vi "KI6221.vi"() -> ()   [LabVIEW 2025] (continued)
                                frame False {
                                }
                                frame True {
                                n821 = while {
                                tunnel: w1577 -> [w1593]
                                tunnel: w1576 -> [w1592]
                                tunnel: w1575 -> [w1588]
                                shift-right: [w1582] -> w1573
                                shift-left: w1574 -> [w1583]
                                tunnel: w1572 -> [w1581]
                                i -> [w1589]
                                stop <- w1586 stop-if-true
                                n822 = Increment(x=w1589) -> (x+1=w1587:i32)
                                n823 = call "VISAreadWrite.vi"("error in (no error)"=w1581, "GPIB INDEX Array"=i32[] [47], "GPIB ARRAY"=w1592, "VISA REFERENCE"=w1593) -> ("error out 15"=→"error out 38":errorcluster, "Read Buffer Array"=w1585:string[])
                                n824 = Greater Or Equal?(x=w1587, y=w1588) -> (x >= y?=w1586:bool)
                                n825 = Index Array(array=w1585, index=1) -> (element=w1579:string)
                                n826 = String Subset(string=w1579, length (rest)=254 ("length (rest)")) -> (substring=w1578:string)  [unwired: 1 in]
                                n827 = Concatenate Strings(w1583, w1578) -> (w1582:string)
                                }
                                }
                                }
                                n828 = String Subset(string=w1541, length (rest)=254 ("length (rest)")) -> (substring=w1540:string)  [unwired: 1 in]
                                n829 = Concatenate Strings(w1540, w1544) -> (w1545:string)
                                n830 = Spreadsheet String To Array(delimiter (Tab)=",", format string="%e", spreadsheet string=w1545, array type (2D Dbl)=dbl[] []) -> (array=w1563:dbl[])
                                n831 = while {
                                tunnel: w1563 -> [w1612]
                                shift-right: [w1611] -> w1556
                                shift-left: string[][] [] -> [w1607]
                                tunnel: w1561 -> [w1600]
                                tunnel: w1560 -> [w1601]
                                tunnel: w1558 -> [w1599]
                                tunnel: w1557 -> [w1598]
                                i -> [w1603]
                                stop <- w1622 stop-if-true
                                w1617 = "," ("delimiter (Tab)")
                                n832 = case shown="0, Default" w1599 {
                                tunnel: w1603 -> [w1625 w1636]
                                tunnel: w1601 -> [w1626 w1634]
                                tunnel: w1600 -> [w1627 w1633]
                                tunnel: [w1623 w1631] -> w1595
                                tunnel: w1598 -> [_ w1628]
                                frame 0, Default {
                                n833 = Multiply(x=w1625, y=w1627) -> (x*y=w1624:dbl)
                                n834 = Add(x=w1626, y=w1624) -> (x+y=w1623:dbl)
                                }
                                frame 1 {
                                n835 = Logarithm Base 10(1:w1634) -> (0:w1630:dbl)
                                n836 = case shown="True" w1628 {
                                tunnel: w1630 -> [w1638 w1639]
                                tunnel: [w1637 w1639] -> w1629
                                frame False {
                                n837 = Negate(x=w1638) -> (-x=w1637:dbl)
                                }
                                frame True {
                                }
                                }
                                n838 = Multiply(x=w1633, y=w1636) -> (x*y=w1632:dbl)
                                n839 = Add(x=w1629, y=w1632) -> (x+y=w1635:dbl)
                                n840 = Power Of 10(x=w1635) -> (10^x=w1631:dbl)
                                }
                                }
                                n841 = Index Array(array=w1612, index=w1603) -> (element=w1605:dbl)
                                n842 = Array Size(array=w1607) -> (size(s)=w1609:i32[])
                                n843 = Index Array(array=w1609, index=0) -> (element=w1606:i32)
                                n844 = Increment(x=w1606) -> (x+1=w1602:i32)
                                n845 = Array Size(array=w1612) -> (size(s)=w1610:i32)
                                n846 = Number To Engineering String(4:w1605) -> (0:w1614:string)  [unwired: 3 in]
                                n847 = Greater Or Equal?(x=w1602, y=w1610) -> (x >= y?=w1622:bool)
                                n848 = Number To Decimal String(number=w1603) -> (decimal integer string=w1616:string)  [unwired: 1 in]
                                n849 = Number To Exponential String(number=w1595, precision (6)=i16 3) -> (E-format string=w1597:string)  [unwired: 2 in]
                                n850 = Fract/Exp String To Number(string=w1597) -> (number=w1594:dbl)  [unwired: 3 in, 1 out]
                                n851 = Divide(x=w1605, y=w1594) -> (x/y=w1604:dbl)
                                n852 = Number To Engineering String(4:w1594) -> (0:w1615:string)  [unwired: 3 in]
                                n853 = Number To Engineering String(4:w1604) -> (0:w1613:string)  [unwired: 3 in]
                                n854 = Concatenate Strings(w1616, w1617, w1615, w1617, w1614, w1617, w1613) -> (w1618:string)
                                n855 = Spreadsheet String To Array(delimiter (Tab)=w1617, format string="%s", spreadsheet string=w1618, array type (2D Dbl)=string[] []) -> (array=w1619:string[])
                                n856 = Insert Into Array(array=w1607, index (row)=w1603, new element=w1619) -> (w1611:string[][])  [unwired: 1 in]
                                }
                                "I Sweep V Measure Data" <- w1556
                                n857 = Array Subset(array=w1556, index (col)=2 ("index"), length (col)=1 ("length")) -> (w1553:string[][])  [unwired: 2 in]
                                n858 = Fract/Exp String To Number(string=w1553) -> (number=w1552:dbl[][])  [unwired: 3 in, 1 out]
                                n859 = Array Max & Min(array=w1552) -> (max value=w1551:dbl)  [unwired: 3 out]
                                n860 = Greater?(x=w1551, y=1e+36) -> (0:w1549:bool)
                                n861 = call "Volt range problem"("Enable"=w1549) -> ()  [unwired: 9 in, 2 out]
                                }
                                }
                                "error out 19" <- w1527
                              }
                            }
                          }
                        }
                        n862 = local write "ABORT SWEEP"(w1425) -> ()
                      }
                      frame True {
                        # "INSTR Missing"
                        n863 = call "LOG error"("Enable"=w1682) -> ()  [unwired: 9 in, 2 out]
                        n864 = Build Array(w1685, w1684, w1683) -> (w1687:bool[])
                        n865 = Boolean Array To Number(Boolean array=w1687) -> (number=w1686:u32)
                        n866 = case shown="3" w1686 {
                          tunnel: w1685 -> [_ w1688 _ _ _ w1691 _ _]
                          tunnel: w1684 -> [_ _ w1689 _ _ _ w1692 _]
                          frame 0, Default {
                          }
                          frame 1 {
                            n867 = call "No 6220/6221 responding"("Enable"=w1688) -> ()  [unwired: 9 in, 2 out]
                          }
                          frame 2 {
                            n868 = call "No 2182/2182A responding"("Enable"=w1689) -> ()  [unwired: 9 in, 2 out]
                          }
                          frame 3 {
                            n869 = call "No Instruments Responding"() -> ()  [unwired: 10 in, 2 out]
                          }
                          frame 4 {
                            n870 = property on="Number of sweep points" class="DigNum (strict)"("Key Focus"=TRUE) -> ()  [unwired: 2 in, 2 out]
                            n871 = call "Too Many Points"() -> ()  [unwired: 10 in, 2 out]
                          }
                          frame 5 {
                            n872 = call "No 6220/6221 responding"("Enable"=w1691) -> ()  [unwired: 9 in, 2 out]
                          }
                          frame 6 {
                            n873 = call "No 2182/2182A responding"("Enable"=w1692) -> ()  [unwired: 9 in, 2 out]
                          }
                          frame 7 {
                            n874 = call "No Instruments Responding"() -> ()  [unwired: 10 in, 2 out]
                          }
                        }
                      }
                    }
                  }
                }
                n875 = local read "enable measure"() -> (w1331:bool)
                n876 = Not Equal?(x="enable measure LAST", y=w1331) -> (x != y?=w1333:bool)
                n877 = case shown="True" w1333 {
                  tunnel: w1331 -> [_ w1358]
                  frame False {
                  }
                  frame True {
                    n878 = case shown="False" w1358 {
                      tunnel: [u8 2 ("Disabled") u8 0 ("Disabled")] -> w1359
                      frame False {
                      }
                      frame True {
                      }
                    }
                    n879 = local write "enable measure LAST"(w1358) -> ()
                    n880 = property on="delta tabs 2" class="TabCtl (strict)"("Disabled"=w1359) -> ()  [unwired: 2 in, 2 out]
                  }
                }
                n881 = Not Equal?(x="X Axis:", y="X Axis: LAST") -> (x != y?=w1338:bool)
                n882 = Not Equal?(x="Y Axis:", y="Y Axis:  LAST") -> (x != y?=w1337:bool)
                n883 = Or(x=w1338, y=w1337) -> (x .or. y?=w1336:bool)
                n884 = case shown="True" w1336 {
                  tunnel: "Y Axis:" -> [_ w1364]
                  tunnel: "X Axis:" -> [_ w1365]
                  frame False {
                  }
                  frame True {
                    n885 = local write "Y Axis:  LAST"(w1364) -> ()
                    n886 = local write "X Axis: LAST"(w1365) -> ()
                    n887 = property on="X Axis:" class="Ring (strict)"() -> ("Strings []"=w1367:string[])  [unwired: 2 in, 2 out]
                    n888 = property on="Y Axis:" class="Ring (strict)"() -> ("Strings []"=w1366:string[])  [unwired: 2 in, 2 out]
                    n889 = local read "I Sweep V Measure Data"() -> (w1371:string[][])
                    n890 = Index Array(array=w1367, index=w1365) -> (element=w1363:string)
                    n891 = Index Array(array=w1366, index=w1364) -> (element=w1362:string)
                    n892 = Index Array(array=w1371, index (col)=w1365) -> (element=w1369:string[])  [unwired: 1 in]
                    n893 = Index Array(array=w1371, index (col)=w1364) -> (element=w1370:string[])  [unwired: 1 in]
                    n894 = Fract/Exp String To Number(string=w1369) -> (number=w1373:dbl[])  [unwired: 3 in, 1 out]
                    n895 = call "Convert to Dynamic Data6"("Array"=w1373) -> ("Dynamic Data Type"=w1374:dynamicdata)  [unwired: 3 in]
                    n896 = Fract/Exp String To Number(string=w1370) -> (number=w1375:dbl[])  [unwired: 3 in, 1 out]
                    n897 = call "Convert to Dynamic Data12"("Array"=w1375) -> ("Dynamic Data Type"=w1368:dynamicdata)  [unwired: 3 in]
                    n898 = call "Build XY Graph4"("Y Input"=w1368, "X Input"=w1374) -> ("XY Graph"=→"I Sweep Graph":cluster{"Y":dbl[], "Y":dbl[]}[])  [unwired: 8 in, 1 out]
                    n899 = property on="I Sweep Graph" class="XYGraph (strict)"("X Scale.Name Label.Text"=w1363, "Y Scale.Name Label.Text"=w1362) -> ()  [unwired: 2 in, 2 out]
                  }
                }
                n900 = local read "ABORT SWEEP"() -> (w1330:bool)
                n901 = Not(x=w1322) -> (.not. x?=w1323:bool)
                n902 = And(x=w1330, y=w1323) -> (x .and. y?=w1324:bool)
                n903 = case shown="True" w1324 {
                  tunnel: w1329 -> [_ w1354]
                  tunnel: w1328 -> [_ w1353]
                  frame False {
                  }
                  frame True {
                    w1350 = TRUE ("Page Selector Visible")
                    n904 = property on="ABORT SWEEP" class="Bool (strict)"("Disabled"=u8 2, "Value"=FALSE ("ABORT SWEEP")) -> ()  [unwired: 2 in, 2 out]
                    n905 = property on="RUN SWEEP" class="Bool"("Disabled"=u8 0) -> ()  [unwired: 2 in, 2 out]
                    n906 = call "VISAreadWrite.vi"("GPIB INDEX Array"=i32[] [36], "GPIB ARRAY"=w1353, "VISA REFERENCE"=w1354) -> ("error out 15"=→"error out 36":errorcluster)  [unwired: 1 in, 1 out]
                    n907 = property on="Basic Source" class="TabCtl (strict)"("Page Selector Visible"=w1350) -> ()  [unwired: 2 in, 2 out]
                    n908 = property on="Main Tabs" class="TabCtl (strict)"("Page Selector Visible"=w1350) -> ()  [unwired: 2 in, 2 out]
                  }
                }
              }
              frame "AC Source" {
                n909 = local write "Source TABS LAST"(w1710) -> ()
                n910 = Not(x=w1702) -> (.not. x?=w1699:bool)
                n911 = And(x="RUN 2", y=w1699) -> (x .and. y?=w1701:bool)
                n912 = local write "waveform tabs 2"("Waveform Type") -> ()
                n913 = local read "6220 VISA"() -> (w1707:refnum<visa-resource-name>)
                n914 = local read "GPIB Array"() -> (w1706:string[])
                n915 = case shown="True" w1701 {
                  tunnel: "Waveform Type" -> [_ w1721]
                  tunnel: w1706 -> [_ w1786]
                  tunnel: w1707 -> [_ w1785]
                  tunnel: [FALSE w1765] -> w1703
                  frame False {
                  }
                  frame True {
                    w1766 = u8 2 ("Disabled")
                    w1767 = 2.0 ("y")
                    # "amplitude"
                    # "offset"
                    # "NOT 6221"
                    n916 = property on="RUN 2" class="Bool"("Disabled"=u8 2) -> ()  [unwired: 2 in, 2 out]
                    n917 = call "VISAreadWrite.vi"("GPIB INDEX Array"=i32[] [0], "GPIB ARRAY"=w1786, "VISA REFERENCE"=w1785) -> ("error out 15"=→"error out 22":errorcluster, "Read Buffer Array"=w1790:string[])  [unwired: 1 in]
                    n918 = property on="Waveform Type" class="Ring (strict)"("Disabled"=w1766) -> ()  [unwired: 2 in, 2 out]
                    n919 = property on="waveform tabs 2" class="TabCtl (strict)"("Disabled"=w1766) -> ()  [unwired: 2 in, 2 out]
                    n920 = Add(x="Ramp from: (Amps)", y="Ramp to: (Amps)") -> (x+y=w1770:dbl)
                    n921 = Subtract(x="Ramp from: (Amps)", y="Ramp to: (Amps)") -> (x-y=w1768:dbl)
                    n922 = Index Array(array=w1790, index=1) -> (element=w1792:string)
                    n923 = Divide(x=w1770, y=w1767) -> (x/y=w1764:dbl)
                    n924 = property on="STOP 2" class="Bool"("Disabled"=u8 0) -> ()  [unwired: 2 in, 2 out]
                    n925 = Divide(x=w1768, y=w1767) -> (x/y=w1769:dbl)
                    n926 = Equal?(x="Ramp from: (Amps)", y="Ramp to: (Amps)") -> (x = y?=w1720:bool)
                    n927 = Absolute Value(x=w1769) -> (abs(x)=w1763:dbl)
                    n928 = Match Pattern(string=w1792, regular expression="MODEL 6221") -> (offset past match=w1789:i32)  [unwired: 1 in, 3 out]
                    n929 = Equal?(x=w1789, y=-1) -> (x = y?=w1727:bool)
                    n930 = property on="Voltage\n Compliance" class="DigNum (strict)"("Disabled"=w1766) -> ()  [unwired: 2 in, 2 out]
                    n931 = Number To Exponential String(number="Duty Cycle (%)") -> (E-format string=w1778:string)  [unwired: 3 in]
                    n932 = Number To Exponential String(number=w1764) -> (E-format string=w1780:string)  [unwired: 3 in]
                    n933 = Number To Exponential String(number=w1763) -> (E-format string=w1779:string)  [unwired: 3 in]
                    n934 = property on="Signal Repetition \nFrequency (Hz)" class="DigNum (strict)"("Disabled"=w1766) -> ()  [unwired: 2 in, 2 out]
                    n935 = Equal?(x=w1721, y=0) -> (x = y?=w1722:bool)
                    n936 = And(x=w1720, y=w1722) -> (x .and. y?=w1719:bool)
                    n937 = Add(x="Offset (Amps)", y="Amplitude (Amps)") -> (x+y=w1756:dbl)
                    n938 = Subtract(x="Offset (Amps)", y="Amplitude (Amps)") -> (x-y=w1755:dbl)
                    n939 = Add(x=w1764, y=w1763) -> (x+y=w1762:dbl)
                    n940 = Subtract(x=w1764, y=w1763) -> (x-y=w1761:dbl)
                    n941 = Greater?(x=w1756, y=0.105) -> (0:w1751:bool)
                    n942 = Less?(x=w1755, y=-0.105) -> (x < y?=w1752:bool)
                    n943 = Greater?(x=w1762, y=0.105) -> (0:w1740:bool)
                    n944 = Less?(x=w1761, y=-0.105) -> (x < y?=w1758:bool)
                    n945 = Or(x=w1751, y=w1752) -> (x .or. y?=w1732:bool)
                    n946 = Number To Exponential String(number="Amplitude (Amps)") -> (E-format string=w1777:string)  [unwired: 3 in]
                    n947 = Number To Exponential String(number="Duty Cycle (%)") -> (E-format string=w1775:string)  [unwired: 3 in]
                    n948 = Number To Exponential String(number="Offset (Amps)") -> (E-format string=w1776:string)  [unwired: 3 in]
                    n949 = Or(x=w1740, y=w1758) -> (x .or. y?=w1734:bool)
                    n950 = Equal?(x=w1721, y=0) -> (x = y?=w1733:bool)
                    n951 = And(x=w1734, y=w1733) -> (x .and. y?=w1730:bool)
                    n952 = Equal?(x=w1721, y=1) -> (x = y?=w1731:bool)
                    n953 = And(x=w1732, y=w1731) -> (x .and. y?=w1729:bool)
                    n954 = Add(x="Offset (Amps)", y="Amplitude (Amps)") -> (x+y=w1750:dbl)
                    n955 = Subtract(x="Offset (Amps)", y="Amplitude (Amps)") -> (x-y=w1749:dbl)
                    n956 = Greater?(x=w1750, y=0.105) -> (0:w1745:bool)
                    n957 = Less?(x=w1749, y=-0.105) -> (x < y?=w1746:bool)
                    n958 = Or(x=w1745, y=w1746) -> (x .or. y?=w1735:bool)
                    n959 = Number To Exponential String(number="Offset (Amps)") -> (E-format string=w1773:string)  [unwired: 3 in]
                    n960 = Number To Exponential String(number="Amplitude (Amps)") -> (E-format string=w1774:string)  [unwired: 3 in]
                    n961 = Number To Exponential String(number="Voltage\n Compliance") -> (E-format string=w1771:string)  [unwired: 3 in]
                    n962 = Number To Exponential String(number="Signal Repetition \nFrequency (Hz)") -> (E-format string=w1772:string)  [unwired: 3 in]
                    n963 = Equal?(x=w1721, y=2) -> (x = y?=w1736:bool)
                    n964 = And(x=w1735, y=w1736) -> (x .and. y?=w1728:bool)
                    n965 = Compound Arithmetic op=OR(w1730, w1729, w1728) -> (w1726:bool)
                    n966 = Compound Arithmetic op=OR(w1727, w1726, w1719) -> (w1757:bool)
                    n967 = case shown="True" w1757 {
                      tunnel: w1721 -> [w1826 _]
                      tunnel: w1786 -> [w1825 _]
                      tunnel: w1785 -> [w1824 _]
                      tunnel: w1780 -> [w1808 _]
                      tunnel: w1779 -> [w1807 _]
                      tunnel: w1778 -> [w1806 _]
                      tunnel: w1777 -> [w1805 _]
                      tunnel: w1776 -> [w1804 _]
                      tunnel: w1775 -> [w1803 _]
                      tunnel: w1774 -> [w1802 _]
                      tunnel: w1773 -> [w1801 _]
                      tunnel: w1772 -> [w1800 _]
                      tunnel: w1771 -> [w1799 _]
                      tunnel: [FALSE TRUE] -> w1765
                      tunnel: w1727 -> [_ w1834]
                      tunnel: w1726 -> [_ w1833]
                      tunnel: w1719 -> [_ w1832]
                      frame False {
                        w1797 = FALSE ("Page Selector Visible")
                        n968 = case shown="2" w1826 {
                          tunnel: [i32[] [39] ("GPIB INDEX Array") i32[] [40] ("GPIB INDEX Array") i32[] [41] ("GPIB INDEX Array")] -> w1827
                          frame 0, Default {
                          }
                          frame 1 {
                          }
                          frame 2 {
                          }
                        }
                        n969 = local read "Setup String"() -> (w1809:string)
                        n970 = Insert Into Array(array=string[] [] ("Replace Array"), new element=w1809) -> (w1812:string[])  [unwired: 1 in]
                        n971 = Insert Into Array(array=w1812, new element=w1808) -> (w1813:string[])  [unwired: 1 in]
                        n972 = property on="Basic Source" class="TabCtl (strict)"("Page Selector Visible"=w1797) -> ()  [unwired: 2 in, 2 out]
                        n973 = property on="Main Tabs" class="TabCtl (strict)"("Page Selector Visible"=w1797) -> ()  [unwired: 2 in, 2 out]
                        n974 = Insert Into Array(array=w1813, new element=w1807) -> (w1814:string[])  [unwired: 1 in]
                        n975 = Insert Into Array(array=w1814, new element=w1806) -> (w1815:string[])  [unwired: 1 in]
                        n976 = Insert Into Array(array=w1815, new element=w1805) -> (w1816:string[])  [unwired: 1 in]
                        n977 = Insert Into Array(array=w1816, new element=w1804) -> (w1817:string[])  [unwired: 1 in]
                        n978 = Insert Into Array(array=w1817, new element=w1803) -> (w1818:string[])  [unwired: 1 in]
                        n979 = Insert Into Array(array=w1818, new element=w1802) -> (w1819:string[])  [unwired: 1 in]
                        n980 = Insert Into Array(array=w1819, new element=w1801) -> (w1820:string[])  [unwired: 1 in]
                        n981 = Insert Into Array(array=w1820, new element=w1800) -> (w1821:string[])  [unwired: 1 in]
                        n982 = Insert Into Array(array=w1821, new element=w1799) -> (w1810:string[])  [unwired: 1 in]
                        n983 = call "VisaVarReplace.vi"("Replace Array"=w1810, "Search Array"=string[] ["<SETUPSTRING>", "<RAMPOFFSET>", "<RAMPAMPLITUDE>", "<RAMPDUTYCYCLE>", "<SQUAREAMPLITUDE>", "<SQUAREOFFSET>", "<SQUAREDUTYCYCLE>", "<SINEAMPLITUDE>", "<SINEOFFSET>", "<FREQUENCY>", "<ACCOMPLIANCE>"], "GPIB Array"=w1825) -> ("GPIB Array OUT"=w1828:string[])
                        n984 = call "VISAreadWrite.vi"("GPIB INDEX Array"=w1827, "GPIB ARRAY"=w1828, "VISA REFERENCE"=w1824) -> ("error out 15"=→"error out 31":errorcluster)  [unwired: 1 in, 1 out]
                      }
                      frame True {
                        n985 = call "No 6221 responding"("Enable"=w1834) -> ()  [unwired: 9 in, 2 out]
                        n986 = call "Current out of range error"("Enable"=w1833) -> ()  [unwired: 9 in, 2 out]
                        n987 = call "Ramp start and stop are equal"("Enable"=w1832) -> ()  [unwired: 9 in, 2 out]
                      }
                    }
                  }
                }
                n988 = Or(x="STOP 2", y=w1703) -> (x .or. y?=w1704:bool)
                n989 = And(x=w1704, y=w1699) -> (x .and. y?=w1700:bool)
                n990 = case shown="True" w1700 {
                  tunnel: w1707 -> [_ w1716]
                  tunnel: w1706 -> [_ w1715]
                  frame False {
                  }
                  frame True {
                    w1711 = TRUE ("Page Selector Visible")
                    w1712 = u8 0 ("Disabled")
                    n991 = call "VISAreadWrite.vi"("GPIB INDEX Array"=i32[] [10], "GPIB ARRAY"=w1715, "VISA REFERENCE"=w1716) -> ("error out 15"=→"error out 35":errorcluster)  [unwired: 1 in, 1 out]
                    n992 = property on="STOP 2" class="Bool"("Disabled"=u8 2) -> ()  [unwired: 2 in, 2 out]
                    n993 = property on="RUN 2" class="Bool"("Disabled"=w1712) -> ()  [unwired: 2 in, 2 out]
                    n994 = property on="Waveform Type" class="Ring (strict)"("Disabled"=w1712) -> ()  [unwired: 2 in, 2 out]
                    n995 = property on="waveform tabs 2" class="TabCtl (strict)"("Disabled"=w1712) -> ()  [unwired: 2 in, 2 out]
                    n996 = property on="Signal Repetition \nFrequency (Hz)" class="DigNum (strict)"("Disabled"=w1712) -> ()  [unwired: 2 in, 2 out]
                    n997 = property on="Voltage\n Compliance" class="DigNum (strict)"("Disabled"=w1712) -> ()  [unwired: 2 in, 2 out]
                    n998 = property on="Basic Source" class="TabCtl (strict)"("Page Selector Visible"=w1711) -> ()  [unwired: 2 in, 2 out]
                    n999 = property on="Main Tabs" class="TabCtl (strict)"("Page Selector Visible"=w1711) -> ()  [unwired: 2 in, 2 out]
                  }
                }
              }
            }
          }
          frame "Advanced Operation" {
            n1000 = case shown="\"Delta Mode Measurements\", Default" "Advanced Operation Tab" {
              frame "Differential Conductance Measurements" {
                w1852 = u8 0 ("Disabled")
                w1844 = TRUE
                # "SETS volt range and compliance when in voltage\nmode, enables user in current mode."
                # "REFERENCED, UNCONNECTED TERMINALS"
                # "UPDATE VOLTAGE OR CURRENT CONTROLS ON GUI"
                # "UPDATE DCON GRAPHS WHEN AXIS OR OFFSET ARE \nCHANGED"
                # "UPDATE 3-D PLOT"
                # "CLEAR SHEET AND GRAPH"
                # "SAVE DATA TO FILE SECTION"
                # "Step source help screen"
                # "THIS CODE IS FOR The step source buttons and options. It runs the EDIT, DELETE, NEW..., and ENABLE states"
                n1001 = case shown="True" "DIFF COND SAVE DATA" {
                  frame False {
                  }
                  frame True {
                    n1002 = File Dialog(4:"KI Data files" ("pattern label"), 5:"Save As" ("button label"), 6:"*.kdf" ("pattern label")) -> (1:w3050:bool, 3:w3049:path)  [unwired: 4 in, 2 out]
                    n1003 = case shown="False" w3050 {
                      tunnel: w3049 -> [w3054 _]
                      frame False {
                        w3058 = "%s" ("format string")
                        n1004 = property on="Differential Conductance Measurement Data" class="Tbl (strict)"() -> ("Column Header Strings[]"=w3059:string[], "Value"=w3060:string[][])  [unwired: 2 in, 2 out]
                        n1005 = Array To Spreadsheet String(array=w3060, 3:w3058) -> (spreadsheet string=w3056:string)  [unwired: 1 in]
                        n1006 = Array To Spreadsheet String(array=w3059, 3:w3058) -> (spreadsheet string=w3057:string)  [unwired: 1 in]
                        n1007 = Concatenate Strings(w3057, w3056) -> (w3055:string)
                        n1008 = call "WriteToFile.vi"("character string"=w3055, "file path (dialog if empty)"=w3054) -> ()  [unwired: 3 in, 1 out]
                      }
                      frame True {
                      }
                    }
                  }
                }
                n1009 = case shown="True" "CLEAR DATA DIFF COND" {
                  frame False {
                  }
                  frame True {
                    n1010 = invoke on="Differential Conductance Measurement Data" class="Table" method="Reinit To Default"() -> ()  [unwired: 3 in, 3 out]
                    n1011 = invoke on="Differential Conductance Graph" class="XYGraph (strict)" method="Reinit To Default"() -> ()  [unwired: 3 in, 3 out]
                    n1012 = invoke on="Differential Conductance Surface Plot" class="AXCont" method="Reinit To Default"() -> ()  [unwired: 3 in, 3 out]
                  }
                }
                n1013 = property on="Advanced Operation Tab" class="TabCtl (strict)"("Page Selector Visible"=w1844) -> ()  [unwired: 2 in, 2 out]
                n1014 = property on="Main Tabs" class="TabCtl (strict)"("Page Selector Visible"=w1844) -> ()  [unwired: 2 in, 2 out]
                n1015 = Not Equal To 0?(x="I want to control my test in terms of:") -> (x != 0?=w1874:bool)
                n1016 = Wait (ms)(milliseconds to wait=u16 400 ("x")) -> ()  [unwired: 1 out]
                n1017 = case shown="True" "HELP" {
                  frame False {
                  }
                  frame True {
                    n1018 = call "Step Source HELP"() -> ()  [unwired: 10 in, 2 out]
                  }
                }
                n1019 = property on="EXIT 2" class="Bool (strict)"("Disabled"=w1852) -> ()  [unwired: 2 in, 2 out]
                n1020 = property on="SAVE 2" class="Bool"("Disabled"=w1852) -> ()  [unwired: 2 in, 2 out]
                n1021 = local read "Differential Conductance Measurement Data"() -> (w1846:string[][])
                n1022 = property on="Horizontal Axis:" class="Ring (strict)"() -> ("Value"=w1886:u16, "Strings []"=w1884:string[])  [unwired: 2 in, 2 out]
                n1023 = property on="Vertical Axis:" class="Ring (strict)"() -> ("Value"=w1885:u16, "Strings []"=w1883:string[])  [unwired: 2 in, 2 out]
                n1024 = Boolean To (0,1)(Boolean=w1874) -> (0, 1=w1877:i16)
                n1025 = local write "V or I DIFF CON tabs"("I want to control my test in terms of:") -> ()
                n1026 = call "Basic Properties.vi"("Differential Conductance Surface Plot"="Differential Conductance Surface Plot", "Int"="Plot style", "plot style"="Transparency (%)") -> ("3D graph out"=w1842:refnum<k7>, "error out"=w1841:errorcluster)  [unwired: 11 in]
                n1027 = local read "Trace offset (% Pk-Pk):"() -> (w1847:dbl)
                n1028 = Multiply(x=2, y=w1877) -> (x*y=w1875:i32)
                n1029 = Not Equal To 0?(x="FILTER") -> (x != 0?=w1838:bool)
                n1030 = call "Basic Properties.vi"("Differential Conductance Surface Plot"=w1842, "fast draw"="Projection", "error in (no error)"=w1841) -> ("3D graph out"=w1843:refnum<k7>, "error out"=→"error out 4":errorcluster)  [unwired: 11 in]
                n1031 = case shown="True" "Plot reset" {
                  tunnel: w1843 -> [_ w1995]
                  frame False {
                  }
                  frame True {
                    n1032 = call "Stub 3d Graph-2.vi"("3D graph out"=w1995) -> ()
                  }
                }
                n1033 = Array Size(array=w1846) -> (size(s)=w1870:i32[])
                n1034 = Equal?(x="Y AXIS LAST -DC", y=w1885) -> (x = y?=w1889:bool)
                n1035 = property on="Define source points with an:" class="Ring (strict)"("Disabled"=w1875) -> ("Value"=w1895:u16)  [unwired: 2 in, 2 out]
                n1036 = Equal?(x="X AXIS LAST -DC", y=w1886) -> (x = y?=w1888:bool)
                n1037 = property on="Repeat Filter Count:" class="DigNum (strict)"("Visible"=w1838) -> ()  [unwired: 2 in, 2 out]
                n1038 = Index Array(array=w1870) -> (element=w1868:i32)  [unwired: 1 in]
                n1039 = Index Array(array=w1870) -> (element=w1869:i32)  [unwired: 1 in]
                n1040 = Equal To 0?(x=w1895) -> (x = 0?=w1873:bool)
                n1041 = Or(x=w1873, y=w1874) -> (x .or. y?=w1872:bool)
                n1042 = Boolean To (0,1)(Boolean=w1872) -> (0, 1=w1894:i16)
                n1043 = Multiply(x=2, y=w1894) -> (x*y=w1893:i32)
                n1044 = property on="Resistance in Ohms" class="DigNum (strict)"("Disabled"=w1893) -> ()  [unwired: 2 in, 2 out]
                n1045 = Equal?(x=w1847, y="OFFSET DC LAST") -> (x = y?=w1864:bool)
                n1046 = Add(x=w1869, y=w1868) -> (x+y=w1867:i32)
                n1047 = Compound Arithmetic op=AND(w1888, w1889, w1864) -> (w1887:bool)
                n1048 = Equal To 0?(x=w1867) -> (x = 0?=w1865:bool)
                n1049 = Or(x=w1887, y=w1865) -> (x .or. y?=w1866:bool)
                n1050 = case shown="True" "RUN DIFF COND" {
                  tunnel: "Differential Conductance Surface Plot" -> [_ w2123]
                  frame False {
                  }
                  frame True {
                    w2117 = TRUE
                    w2114 = FALSE
                    w2150 = "%s" ("format string")
                    w2130 = 0
                    w2131 = 2
                    n1051 = property on="ABORT DIFF COND" class="Bool (strict)"("Value"=FALSE ("ABORT DIFF COND"), "Disabled"=0) -> (error out=w2156:errorcluster)  [unwired: 2 in, 1 out]
                    n1052 = property on="Main Tabs" class="TabCtl (strict)"("Page Selector Visible"=w2114) -> (error out=w2113:errorcluster)  [unwired: 2 in, 1 out]
                    n1053 = property on="Advanced Operation Tab" class="TabCtl (strict)"(error in=w2113, "Page Selector Visible"=w2114) -> (error out=w2132:errorcluster)  [unwired: 1 in, 1 out]
                    n1054 = property on="RUN DIFF COND" class="Bool"(error in=w2132, "Disabled"=u16 2 ("x")) -> (error out=w2135:errorcluster)  [unwired: 1 in, 1 out]
                    n1055 = invoke on="Differential Conductance Measurement Data" class="Table" method="Reinit To Default"(error in=w2135) -> (error out=w2121:errorcluster)  [unwired: 2 in, 2 out]
                    n1056 = property on="Enable \nSTEP SOURCE" class="Bool (strict)"() -> ("Value"=w2151:bool)  [unwired: 2 in, 2 out]
                    n1057 = invoke on="Differential Conductance Surface Plot" class="AXCont" method="Reinit To Default"(error in=w2121) -> (error out=w2124:errorcluster)  [unwired: 2 in, 2 out]
                    n1058 = invoke on="Differential Conductance Graph" class="XYGraph (strict)" method="Reinit To Default"(error in=w2124) -> (error out=w2122:errorcluster)  [unwired: 2 in, 2 out]
                    n1059 = property on="DEMO MODE" class="Bool (strict)"(error in=w2122) -> ("Value"=w2161:bool)  [unwired: 1 in, 2 out]
                    n1060 = property on="Horizontal Axis:" class="Ring (strict)"("Disabled"=w2131) -> ("Value"=w2158:u16, "Strings []"=w2160:string[])  [unwired: 2 in, 2 out]
                    n1061 = property on="Vertical Axis:" class="Ring (strict)"("Disabled"=w2131) -> ("Value"=w2157:u16, "Strings []"=w2159:string[])  [unwired: 2 in, 2 out]
                    n1062 = Index Array(array=w2160, index=w2158) -> (element=w2125:string)
                    n1063 = Index Array(array=w2159, index=w2157) -> (element=w2126:string)
                    n1064 = property on="Trace offset (% Pk-Pk):" class="DigNum (strict)"("Disabled"=w2131) -> ("Value"=w2128:dbl)  [unwired: 2 in, 2 out]
                    n1065 = Divide(x=w2128, y=100.0) -> (x/y=w2129:dbl)
                    n1066 = property on="Differential Conductance Graph" class="XYGraph (strict)"("Y Scale.Name Label.Text"=w2126, "X Scale.Name Label.Text"=w2125) -> ()  [unwired: 2 in, 2 out]
                    n1067 = property on="Current Test File:" class="Path"() -> ("Value"=w2138:path)  [unwired: 2 in, 2 out]
                    n1068 = Equal?(x=w2138, y=path "") -> (x = y?=w2139:bool)
                    n1069 = case shown="False" w2139 {
                      tunnel: w2138 -> [w2163 _]
                      tunnel: [w2162 w2169] -> w2137
                      frame False {
                        n1070 = Path To String(path=w2163) -> (string=w2167:string)
                        n1071 = Search/Split String(string=w2167, search string/char (-)=".") -> (substring before match=w2166:string)  [unwired: 1 in, 2 out]
                        n1072 = Concatenate Strings(w2166, "_dcdata.kdf" ("search string/char (-)")) -> (w2164:string)
                        n1073 = String To Path(string=w2164) -> (path=w2162:path)
                      }
                      frame True {
                        n1074 = property on="Default path" class="Path"() -> ("Value"=w2170:path)  [unwired: 2 in, 2 out]
                        n1075 = Build Path(base path=w2170, name or relative path="DefaultTestFile_dcdata.cfg" ("file path (dialog if empty)")) -> (appended path=w2169:path)
                      }
                    }
                    n1076 = call <vilib>:"Read Lines From File.vi"("convert eol? (no:F)"=TRUE, "file path (dialog if empty)"=w2137, "number of lines (all:-1)"=-1) -> ("line string"=w2148:string)  [unwired: 3 in, 3 out]
                    n1077 = Match Pattern(string=w2148, regular expression="\n") -> (before substring=w2146:string, match substring=w2145:string, after substring=w2143:string)  [unwired: 1 in, 1 out]
                    n1078 = Concatenate Strings(w2146, w2145) -> (w2144:string)
                    n1079 = Spreadsheet String To Array(format string=w2150, spreadsheet string=w2144, array type (2D Dbl)=string[] []) -> ()  [unwired: 1 in, 1 out]
                    n1080 = Spreadsheet String To Array(format string=w2150, spreadsheet string=w2143, array type (2D Dbl)=string[][] []) -> (array=w2136:string[][])  [unwired: 1 in]
                    n1081 = case shown="False" w2161 {
                      tunnel: w2136 -> [_ w2860]
                      tunnel: w2158 -> [_ w2868]
                      tunnel: w2157 -> [_ w2869]
                      tunnel: w2156 -> [w2172 w2851]
                      tunnel: w2151 -> [_ w2867]
                      tunnel: w2129 -> [_ w2854]
                      tunnel: w2123 -> [w2175 w2852]
                      tunnel: [w2172 w2851] -> w2112
                      frame False {
                        # "TEST SETUP ERROR STATES..."
                        # "NOT 6221"
                        n1082 = property on="Start Voltage  (Volts)" class="DigNum (strict)"() -> ("Value"=w2213:dbl)  [unwired: 2 in, 2 out]
                        n1083 = property on="GPIB Array" class="Arr (strict)"() -> ("Value"=w2176:string[])  [unwired: 2 in, 2 out]
                        n1084 = property on="6220 VISA" class="VISAName"() -> ("Value"=w2177:refnum<visa-resource-name>)  [unwired: 2 in, 2 out]
                        n1085 = property on="Current Source \nVoltage Compliance (V)" class="DigNum (strict)"() -> ("Value"=w2211:dbl)  [unwired: 2 in, 2 out]
                        n1086 = property on="I want to control my test in terms of:" class="Ring (strict)"() -> ("Value"=w2210:u16)  [unwired: 2 in, 2 out]
                        n1087 = property on="Select the nanovoltmeter model number:" class="Ring (strict)"() -> ("Value"=w2193:u16)  [unwired: 2 in, 2 out]
                        n1088 = call "VISAreadWrite.vi"("GPIB INDEX Array"=i32[] [0, 13], "GPIB ARRAY"=w2176, "VISA REFERENCE"=w2177) -> ("error out 15"=→"error out 24":errorcluster, "Read Buffer Array"=w2186:string[])  [unwired: 1 in]
                        n1089 = Index Array(array=w2186, index=1) -> (element=w2191:string)
                        n1090 = Index Array(array=w2186, index=3) -> (element=w2185:string)
                        n1091 = Absolute Value(x=w2213) -> (abs(x)=w2174:dbl)
                        n1092 = Not Equal To 0?(x=w2210) -> (x != 0?=w2201:bool)
                        n1093 = Less Or Equal?(x=w2174, y=w2211) -> (x <= y?=w2206:bool)
                        n1094 = Not(x=w2201) -> (.not. x?=w2208:bool)
                        n1095 = Not(x=w2201) -> (.not. x?=w2204:bool)
                        n1096 = Match Pattern(string=w2191, regular expression="MODEL 622") -> (offset past match=w2183:i32)  [unwired: 1 in, 3 out]
                        n1097 = Greater?(x=w2193, y=u16 1 ("x")) -> (0:w2194:bool)
                        n1098 = Decimal String To Number(string=w2185) -> (number=w2184:i32)  [unwired: 2 in, 1 out]
                        n1099 = Equal?(x=w2183, y=-1) -> (x = y?=w2181:bool)
                        n1100 = Not(x=w2206) -> (.not. x?=w2205:bool)
                        n1101 = And(x=w2205, y=w2208) -> (x .and. y?=w2207:bool)
                        n1102 = property on="Stop Voltage (Volts)" class="DigNum (strict)"() -> ("Value"=w2212:dbl)  [unwired: 2 in, 2 out]
                        n1103 = Equal To 0?(x=w2184) -> (x = 0?=w2180:bool)
                        n1104 = Not(x=w2207) -> (.not. x?=w2199:bool)
                        n1105 = Absolute Value(x=w2212) -> (abs(x)=w2173:dbl)
                        n1106 = Less Or Equal?(x=w2173, y=w2211) -> (x <= y?=w2200:bool)
                        n1107 = Not(x=w2200) -> (.not. x?=w2202:bool)
                        n1108 = And(x=w2202, y=w2204) -> (x .and. y?=w2203:bool)
                        n1109 = And(x=w2200, y=w2206) -> (x .and. y?=w2209:bool)
                        n1110 = Or(x=w2209, y=w2201) -> (x .or. y?=w2196:bool)
                        n1111 = Not(x=w2203) -> (.not. x?=w2198:bool)
                        n1112 = Or(x=w2180, y=w2181) -> (x .or. y?=w2178:bool)
                        n1113 = Not(x=w2178) -> (.not. x?=w2179:bool)
                        n1114 = Compound Arithmetic op=AND(w2196, w2194, w2179) -> (w2195:bool)
                        n1115 = case shown="False" w2195 {
                          tunnel: w2199 -> [w2220 _]
                          tunnel: w2198 -> [w2219 _]
                          tunnel: w2194 -> [w2218 _]
                          tunnel: w2181 -> [w2216 _]
                          tunnel: w2180 -> [w2217 _]
                          tunnel: w2177 -> [_ w2232]
                          tunnel: w2176 -> [_ w2231]
                          tunnel: w2175 -> [_ w2230]
                          frame False {
                            n1116 = Not(x=w2216) -> (.not. x?=w2214:bool)
                            n1117 = And(x=w2217, y=w2214) -> (x .and. y?=w2215:bool)
                            n1118 = call "No 6220/6221 found"("Enable"=w2216) -> ()  [unwired: 9 in, 2 out]
                            n1119 = case shown="False" w2219 {
                              frame False {
                                n1120 = One Button Dialog(message="To run a test the absolute value of Stop Voltage (mV) must be\nless than or equal to the Current Source Voltage Compliance. \nChange a value, then click RUN again.") -> (true=w2223:bool)  [unwired: 1 in]
                                n1121 = case shown="False" w2223 {
                                frame False {
                                }
                                frame True, Default {
                                n1122 = property on="Current Source \nVoltage Compliance (V)" class="DigNum (strict)"("Key Focus"=TRUE) -> ()  [unwired: 2 in, 2 out]
                                }
                                }
                              }
                              frame True {
                              }
                            }
                            n1123 = case shown="False" w2220 {
                              frame False {
                                n1124 = One Button Dialog(message="To run a test the absolute value of Start Voltage (mV) must be\nless than or equal to the Current Source Voltage Compliance. \nChange a value, then click RUN again.") -> (true=w2226:bool)  [unwired: 1 in]
                                n1125 = case shown="False" w2226 {
                                frame False {
                                }
                                frame True, Default {
                                n1126 = property on="Current Source \nVoltage Compliance (V)" class="DigNum (strict)"("Key Focus"=TRUE) -> ()  [unwired: 2 in, 2 out]
                                }
                                }
                              }
                              frame True {
                              }
                            }
                            n1127 = case shown="False" w2218 {
                              frame False {
                                n1128 = One Button Dialog(message="To run a differential conductance test, both a current \nsource and a nanovoltmeter must be connected and \nconfigured in the instrument communication panel.") -> (true=w2221:bool)  [unwired: 1 in]
                                n1129 = case shown="False" w2221 {
                                frame False {
                                }
                                frame True, Default {
                                }
                                }
                              }
                              frame True {
                              }
                            }
                            n1130 = call "No 2182"("Enable"=w2215) -> ()  [unwired: 9 in, 2 out]
                          }
                          frame True {
                            (unwired) "Initiating Test. Make certain device is correctly connected\nto the instruments, then click OK. "
                            # "ACTUAL DATA COMMUNICATION"
                            n1131 = case shown="True" "Case Constant\n(See Context Help) 4" {
                              tunnel: w2232 -> [_ w2311]
                              tunnel: w2231 -> [_ w2310]
                              tunnel: w2230 -> [_ w2302]
                              frame False {
                              }
                              frame True {
                                w2250 = 1e-09
                                w2235 = TRUE
                                w2238 = FALSE
                                # "SET 3-D GRAPH TAB to ENABLE based on # sweeps."
                                # "CREATE DATA SHEET HEADER"
                                # "CHECK FOR STEP SOURCE\nCONNECTED..."
                                n1132 = property on="Start Current (Amps)" class="DigNum (strict)"() -> ("Value"=w2331:dbl)  [unwired: 2 in, 2 out]
                                n1133 = property on="Delay (settle time in mS)" class="DigNum (strict)"() -> ("Value"=w2252:dbl)  [unwired: 2 in, 2 out]
                                n1134 = property on="Voltage Measure Range" class="Ring (strict)"() -> ("Value"=w2307:dbl)  [unwired: 2 in, 2 out]
                                n1135 = property on="Current Source \nVoltage Compliance (V)" class="DigNum (strict)"() -> ("Value"=w2306:dbl)  [unwired: 2 in, 2 out]
                                n1136 = property on="Stop Current (Amps)" class="DigNum (strict)"() -> ("Value"=w2330:dbl)  [unwired: 2 in, 2 out]
                                n1137 = property on="Number of sweep points" class="DigNum (strict)"() -> ("Value"=w2329:i32)  [unwired: 2 in, 2 out]
                                n1138 = property on="FILTER" class="Ring (strict)"() -> ("Value"=w2243:u16)  [unwired: 2 in, 2 out]
                                n1139 = Divide(x=w2252, y=1000.0) -> (x/y=w2253:dbl)
                                n1140 = Number To Exponential String(number=w2253) -> (E-format string=w2305:string)  [unwired: 3 in]
                                n1141 = Number To Exponential String(number=w2307) -> (E-format string=w2262:string)  [unwired: 3 in]
                                n1142 = property on="Number of sweep points" class="DigNum (strict)"() -> ("Value"=w2326:i32)  [unwired: 2 in, 2 out]
                                n1143 = property on="Measurement Integration (NPLCs)" class="DigNum (strict)"() -> ("Value"=w2233:dbl)  [unwired: 2 in, 2 out]
                                n1144 = property on="Repeat Filter Count:" class="DigNum (strict)"() -> ("Value"=w2242:i32)  [unwired: 2 in, 2 out]
                                n1145 = Number To Decimal String(number=w2242) -> (decimal integer string=w2241:string)  [unwired: 1 in]
                                n1146 = property on="Start Voltage  (Volts)" class="DigNum (strict)"() -> ("Value"=w2328:dbl)  [unwired: 2 in, 2 out]
                                n1147 = property on="DIFF COND DAMPING" class="Bool (strict)"() -> ("Value"=w2309:bool)  [unwired: 2 in, 2 out]
                                n1148 = property on="Define source points with an:" class="Ring (strict)"() -> ("Value"=w2332:u16)  [unwired: 2 in, 2 out]
                                n1149 = Number To Exponential String(number=w2306) -> (E-format string=w2263:string)  [unwired: 3 in]
                                n1150 = property on="Stop Voltage (Volts)" class="DigNum (strict)"() -> ("Value"=w2327:dbl)  [unwired: 2 in, 2 out]
                                n1151 = property on="Advanced Operation Tab" class="TabCtl (strict)"("Page Selector Visible"=w2238) -> (error out=w2239:errorcluster)  [unwired: 2 in, 1 out]
                                n1152 = Boolean To (0,1)(Boolean=w2309) -> (0, 1=w2308:i16)
                                n1153 = Concatenate Strings("VERIFY:", "\n", "ENTER1024" ("string")) -> (w2319:string)
                                n1154 = Insert Into Array(array=string[] [], new element=w2319) -> (w2324:string[])  [unwired: 1 in]
                                n1155 = Insert Into Array(array=w2324, new element="CONFIGURE:") -> (w2323:string[])  [unwired: 1 in]
                                n1156 = case shown="0" w2243 {
                                tunnel: ["1" "0"] -> w2304
                                frame 1, Default {
                                }
                                frame 0 {
                                }
                                }
                                n1157 = Insert Into Array(array=string[] [], new element=w2263) -> (w2268:string[])  [unwired: 1 in]
                                n1158 = Number To Decimal String(number=w2308) -> (decimal integer string=w2260:string)  [unwired: 1 in]
                                n1159 = Insert Into Array(array=w2268, new element=w2260) -> (w2267:string[])  [unwired: 1 in]
                                n1160 = Insert Into Array(array=w2267, new element=w2262) -> (w2266:string[])  [unwired: 1 in]
                                n1161 = Number To Exponential String(number=w2233) -> (E-format string=w2261:string)  [unwired: 3 in]
                                n1162 = property on="step VISA" class="VISAName"() -> ("Value"=w2278:refnum<visa-resource-name>)  [unwired: 2 in, 2 out]
                                n1163 = property on="Main Tabs" class="TabCtl (strict)"(error in=w2239, "Page Selector Visible"=w2238) -> (error out=w2240:errorcluster)  [unwired: 1 in, 1 out]
                                n1164 = property on="Number of steps" class="DigNum (strict)"(error in=w2240) -> (error out=w2333:errorcluster, "Value"=w2335:i32, "Disabled"=w2273:u8)  [unwired: 1 in, 1 out]
                                n1165 = property on="I want to control my test in terms of:" class="Ring (strict)"(error in=w2333) -> ("Value"=w2334:u16)  [unwired: 1 in, 2 out]
                                n1166 = Insert Into Array(array=w2266, new element=w2261) -> (w2265:string[])  [unwired: 1 in]
                                n1167 = Equal?(x="VERIFY:", y="") -> (x = y?=w2317:bool)
                                n1168 = Insert Into Array(array=w2265, new element="1e-9" ("new element/subarray")) -> (w2264:string[])  [unwired: 1 in]
                                n1169 = Number To Decimal String(number="DELAY in mS") -> (decimal integer string=w2270:string)  [unwired: 1 in]
                                n1170 = property on="INSTRUMENT NAME:" class="Str"() -> ("Value"=w2300:string)  [unwired: 2 in, 2 out]
                                n1171 = Concatenate Strings("GO TO LEVEL:                *NOTE - MUST include <LEVEL>", "\n", "WAIT" ("string"), w2270) -> (w2315:string)
                                n1172 = Insert Into Array(array=w2323, new element=w2315) -> (w2322:string[])  [unwired: 1 in]
                                n1173 = Insert Into Array(array=w2322, new element="DEACTIVATE:") -> (w2277:string[])  [unwired: 1 in]
                                n1174 = Equal?(x=w2300, y="Window Pop-up") -> (x = y?=w2275:bool)
                                n1175 = Not(x=w2275) -> (.not. x?=w2274:bool)
                                n1176 = Equal?(x=w2273, y=u8 0) -> (x = y?=w2276:bool)
                                n1177 = And(x=w2276, y=w2274) -> (x .and. y?=w2271:bool)
                                n1178 = case shown="0, Default" w2273 {
                                tunnel: w2335 -> [w2380 _]
                                tunnel: [w2380 1 ("Value")] -> w2285
                                tunnel: w2277 -> [w2374 _]
                                tunnel: w2278 -> [w2375 _]
                                tunnel: [w2377 w2404] -> w2312
                                tunnel: [w2372 w2404] -> w2313
                                tunnel: w2317 -> [w2376 _]
                                tunnel: w2275 -> [w2371 _]
                                frame 0, Default {
                                n1179 = case shown="False" w2371 {
                                tunnel: w2376 -> [w2385 _]
                                tunnel: w2375 -> [w2382 _]
                                tunnel: w2374 -> [w2381 _]
                                frame False {
                                n1180 = case shown="False" w2385 {
                                tunnel: [w2395 FALSE] -> w2384
                                tunnel: w2382 -> [w2394 _]
                                tunnel: w2381 -> [w2393 _]
                                tunnel: [w2392 errorcluster {"status"=FALSE, "code"=0, "source"=""} ("error out 15")] -> w2383
                                frame False {
                                # "NOT STEP"
                                n1181 = call "VISAreadWrite.vi"("GPIB INDEX Array"=i32[] [0], "GPIB ARRAY"=w2393, "VISA REFERENCE"=w2394) -> ("error out 15"=w2392:errorcluster, "Read Buffer Array"=w2400:string[])  [unwired: 1 in]
                                n1182 = Index Array(array=w2400, index=1) -> (element=w2397:string)
                                n1183 = Match Pattern(string=w2397, regular expression="RESPONSE STRING:") -> (offset past match=w2401:i32)  [unwired: 1 in, 3 out]
                                n1184 = Equal?(x=w2401, y=-1) -> (x = y?=w2395:bool)
                                }
                                frame True {
                                }
                                }
                                n1185 = case shown="False" w2384 {
                                tunnel: w2383 -> [w2389 _]
                                tunnel: w2382 -> [w2388 _]
                                tunnel: w2381 -> [w2387 _]
                                frame False {
                                n1186 = call "VISAreadWrite.vi"("error in (no error)"=w2389, "GPIB INDEX Array"=i32[] [1], "GPIB ARRAY"=w2387, "VISA REFERENCE"=w2388) -> ("error out 15"=w2386:errorcluster)  [unwired: 1 out]
                                n1187 = case shown="Error" w2386 {
                                frame No Error {
                                }
                                frame Error {
                                n1188 = call "STEP SOURCE ERROR MESS2"() -> ()  [unwired: 10 in, 2 out]
                                }
                                }
                                }
                                frame True {
                                n1189 = call "STEP SOURCE ERROR MESS"() -> ()  [unwired: 10 in, 2 out]
                                }
                                }
                                }
                                frame True {
                                }
                                }
                                n1190 = property on="Stop Level" class="DigNum (strict)"() -> ("Value"=w2373:dbl)  [unwired: 2 in, 2 out]
                                n1191 = property on="Start Level" class="DigNum (strict)"() -> ("Value"=w2372:dbl)  [unwired: 2 in, 2 out]
                                n1192 = Decrement(x=w2380) -> (x-1=w2379:i32)
                                n1193 = Subtract(x=w2373, y=w2372) -> (x-y=w2378:dbl)
                                n1194 = Divide(x=w2378, y=w2379) -> (x/y=w2377:dbl)
                                }
                                frame 2 {
                                w2404 = 0.0 ("Value")
                                }
                                }
                                n1195 = while {
                                tunnel: w2285 -> [w2463]
                                tunnel: w2334 -> [w2460]
                                tunnel: w2273 -> [w2459]
                                tunnel: w2332 -> [w2458]
                                tunnel: w2331 -> [w2457]
                                tunnel: w2330 -> [w2456]
                                tunnel: w2329 -> [w2455]
                                tunnel: w2328 -> [w2454]
                                tunnel: w2327 -> [w2453]
                                tunnel: w2326 -> [w2452]
                                tunnel: w2277 -> [w2450]
                                tunnel: w2278 -> [w2449]
                                tunnel: w2312 -> [w2448]
                                shift-right: [w2447] -> _
                                shift-left: w2313 -> [w2435]
                                tunnel: w2311 -> [w2424]
                                tunnel: w2310 -> [w2423]
                                tunnel: w2305 -> [w2443]
                                tunnel: w2263 -> [w2442]
                                tunnel: w2260 -> [w2441]
                                tunnel: w2262 -> [w2440]
                                tunnel: w2261 -> [w2439]
                                tunnel: w2304 -> [w2438]
                                tunnel: w2241 -> [w2437]
                                tunnel: w2242 -> [w2434]
                                shift-right: [w2433] -> w2244
                                shift-left: string[][] [] -> [w2432]
                                shift-right: [w2429] -> _
                                shift-left: cluster{dbl[], dbl[], dbl[]} {[], [], []} -> [w2428]
                                tunnel: w2302 -> [w2427]
                                tunnel: w2275 -> [w2426]
                                tunnel: [w2425] -> w2236
                                shift-right: [w2420] -> _
                                shift-left: w2264 -> [w2422]
                                tunnel: [w2418] -> w2258
                                tunnel: [w2417] -> w2254
                                shift-right: [w2407] -> _
                                shift-left: w2250 -> [w2413]
                                shift-right: [w2408] -> _
                                shift-left: w2250 -> [w2409]
                                tunnel: [w2411] -> w2234
                                tunnel: w2233 -> [w2406]
                                i -> [w2430]
                                stop <- w2451 stop-if-true
                                n1196 = flat-sequence {
                                tunnel: [w2473] -> w2461
                                tunnel: w2460 -> [w2473]
                                tunnel: w2459 -> [w2472]
                                tunnel: w2450 -> [w2471]
                                tunnel: w2449 -> [w2470]
                                tunnel: w2435 -> [w2469]
                                tunnel: w2448 -> [w2468]
                                tunnel: [w2467] -> w2447
                                tunnel: w2430 -> [w2465]
                                tunnel: w2426 -> [w2464]
                                tunnel: w2461 -> [w2522]
                                tunnel: w2458 -> [w2521]
                                tunnel: w2457 -> [w2520]
                                tunnel: w2456 -> [w2519]
                                tunnel: w2455 -> [w2518]
                                tunnel: w2454 -> [w2517]
                                tunnel: w2453 -> [w2516]
                                tunnel: w2452 -> [w2515]
                                tunnel: [w2507] -> w2446
                                tunnel: [w2506] -> w2445
                                tunnel: [w2514] -> w2444
                                tunnel: [w2513] -> w2436
                                tunnel: w2434 -> [_]
                                tunnel: w2424 -> [w2512]
                                tunnel: w2423 -> [w2511]
                                tunnel: w2422 -> [w2510]
                                tunnel: [w2509] -> w2421
                                tunnel: [w2508] -> w2419
                                tunnel: [w2507] -> w2415
                                tunnel: [w2506] -> w2414
                                tunnel: w2409 -> [w2505]
                                tunnel: w2413 -> [w2504]
                                tunnel: [w2624] -> w2412
                                tunnel: w2424 -> [w2604]
                                tunnel: w2423 -> [w2623]
                                tunnel: w2446 -> [w2613]
                                tunnel: w2445 -> [w2610]
                                tunnel: w2444 -> [w2599]
                                tunnel: w2443 -> [w2632]
                                tunnel: w2442 -> [w2631]
                                tunnel: w2441 -> [w2630]
                                tunnel: w2440 -> [w2629]
